vi "Add SPI Engine to Project and Lib.vi"(7 "Number of SPI Buses in":i32, 8 "error in (no error)":errorcluster, 9 "LabVIEW Project to Script":path, 10 "Curent Bus Path":path, 11 "Replacement VI for SPI Engine":path) -> (0 "error out":errorcluster)   [LabVIEW 2014, in "SPI Engine Scripting.lvlib"]
uses:
  SPI Engine Scripting.lvlib
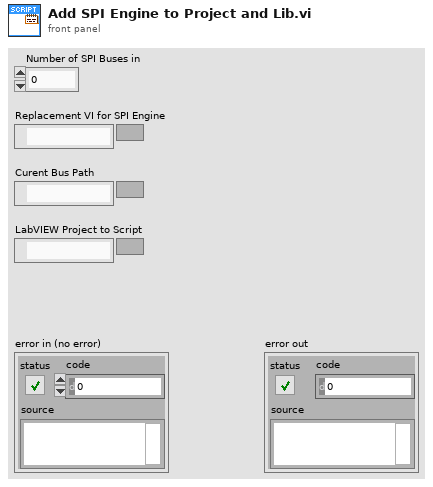
[diagram p1: front panel]
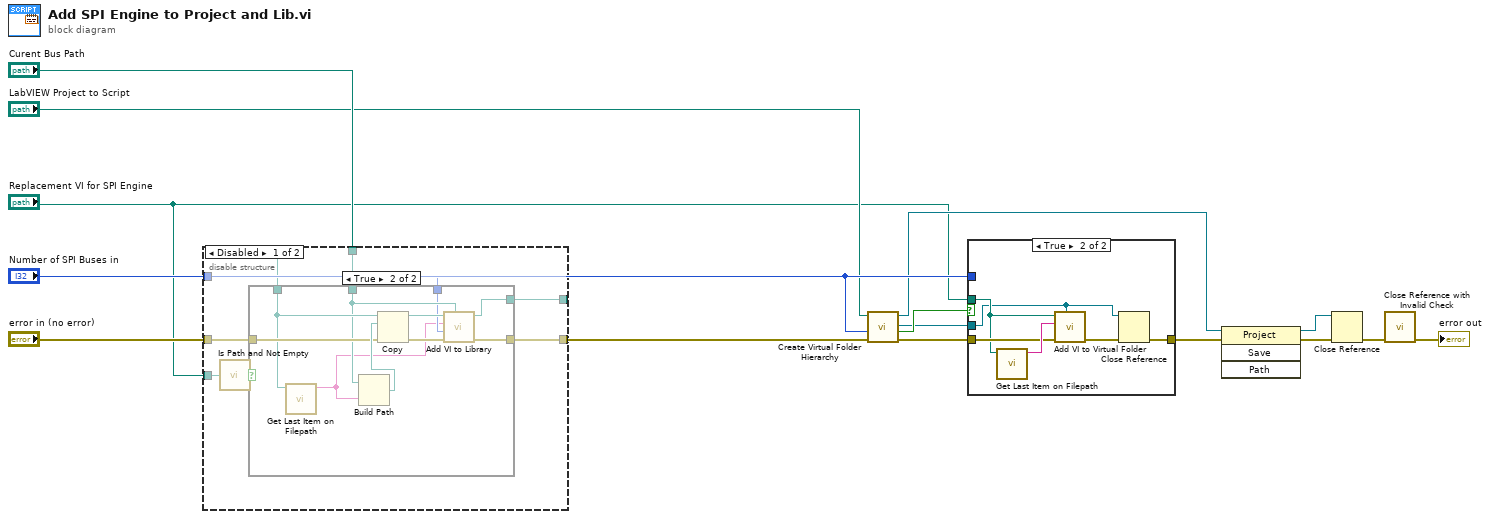
[diagram p0: block diagram]
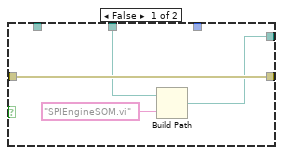
[diagram p2: hidden frame]
diagram:
  n1 = disable-structure shown="Disabled" {
    disable-tunnel: [w22 _] -> _
    disable-tunnel: "Number of SPI Buses in" -> [w21 _]
    disable-tunnel: "Curent Bus Path" -> [w19 _]
    disable-tunnel: "Replacement VI for SPI Engine" -> [w18 _]
    disable-tunnel: [w17 _] -> w13
    disable-tunnel: "error in (no error)" -> [w16 _]
    frame Disabled {
      n2 = call <vilib>:"Is Path and Not Empty.vi"("path"=w18) -> ("Is Path and Not Empty?"=w20:bool)  [unwired: 4 in]
      n3 = case shown="True" w20 {
        tunnel: w16 -> [w26 w33]
        tunnel: [w26 w32] -> w17
        tunnel: w18 -> [_ w31]
        tunnel: w19 -> [w24 w30]
        tunnel: w21 -> [_ w29]
        tunnel: [w23 w27] -> w22
        frame False {
          n4 = Build Path(base path=w24, name or relative path="SPIEngineSOM.vi" ("VI to Code Relative Path")) -> (appended path=w23:path)
        }
        frame True {
          n5 = call "Get Last Item on Filepath.vi"("Replacement VI for SPI Engine"=w31) -> ("String"=w28:string)  [unwired: 10 in]
          n6 = Build Path(base path=w30, name or relative path=w28) -> (appended path=w34:path)
          n7 = Copy(8:w33, 10:w34, 11:w31) -> (0:w36:errorcluster, 3:w35:path)  [unwired: 2 in, 1 out]
          n8 = call "Add VI to Library.vi"("Current Bus Path"=w30, "error in"=w36, "Bus Number"=w29, "VI Name"=w28, "Path to new VI"=w35) -> ("error out"=w32:errorcluster, "Path to new IO Node"=w27:path)  [unwired: 5 in]
        }
      }
    }
    frame Enabled {
    }
  }
  n9 = call "Create Virtual Folder Hierarchy.vi"("error in"=w13, "Bus Number"="Number of SPI Buses in", "Path to Project"="LabVIEW Project to Script") -> ("error out"=w5:errorcluster, "FPGA Target Found"=w9:bool, "New Virtual Folder"=w7:refnum<vi>, "Project:Open"=w4:refnum<vi>)  [unwired: 5 in]
  n10 = case shown="True" w9 {
    tunnel: w5 -> [w37 w41]
    tunnel: "Number of SPI Buses in" -> [_ _]
    tunnel: [w37 w38] -> w6
    tunnel: w7 -> [_ w39]
    tunnel: "Replacement VI for SPI Engine" -> [_ w40]
    frame False {
    }
    frame True {
      n11 = call "Get Last Item on Filepath.vi"("Replacement VI for SPI Engine"=w40) -> ("String"=w42:string)  [unwired: 10 in]
      n12 = call "Add VI to Virtual Folder.vi"("Virtual Folder"=w39, "error in"=w41, "VI Name"=w42, "Path to VI"=w40) -> ("error out"=w43:errorcluster)  [unwired: 5 in, 2 out]
      n13 = Close Reference(reference=w39, error in (no error)=w43) -> (error out=w38:errorcluster)
    }
  }
  n14 = invoke class="Project" method="Save"(reference=w4, error in=w6) -> (reference out=w11:refnum<vi>, error out=w10:errorcluster)  [unwired: 2 in, 2 out]
  n15 = Close Reference(reference=w11, error in (no error)=w10) -> (error out=w2:errorcluster)
  n16 = call "Close Reference with Invalid Check.vi"("error in (no error)"=w2) -> ("error out"=→"error out":errorcluster)  [unwired: 10 in]
